vi "WSVCAP SHL Host LL Interface Manage Instance IDs.vi"(6 "Operation":T2, 8 "error in (no error)":errorcluster, 11 "FPGA":T3) -> (0 "error out":errorcluster, 3 "Instance IDs":T1)   [LabVIEW 2012]
uses:
  Type Defs/WSVCAP SHL I2C FPGA Enum.ctl
  user.lib/Utilities/Type Defs/MISC Instance Manager Operation.ctl
  Type Defs/WSVCAP SHL FPGA Interface Instance Ref Cluster.ctl
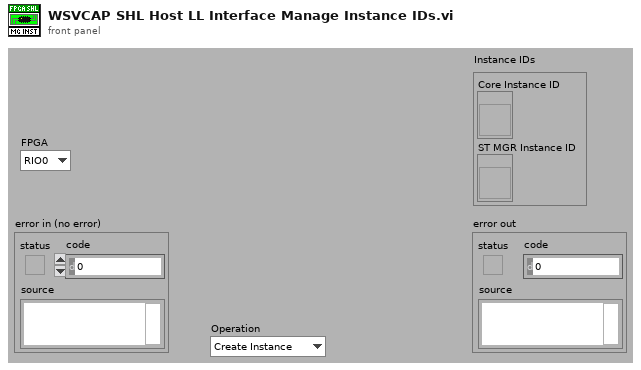
[diagram p1: front panel]
types:
  T1 = typedef "WSVCAP SHL FPGA Interface Instance Ref Cluster.ctl" = cluster{"Core Instance ID":refnum<vi>, "ST MGR Instance ID":refnum<vi>}
  T2 = typedef "MISC Instance Manager Operation.ctl" = enum16{"Create Instance", "Get Instance ID"}
  T3 = typedef "WSVCAP SHL I2C FPGA Enum.ctl" = enum16{"RIO0", "RIO1"}
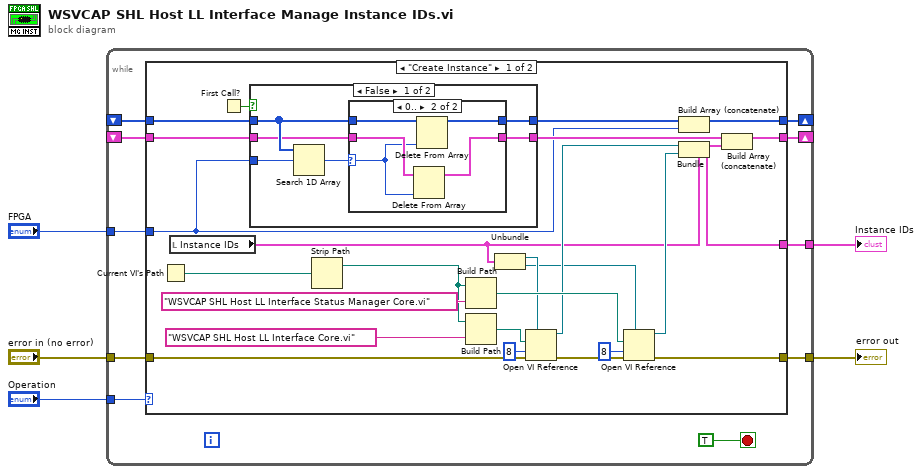
[diagram p0: block diagram]
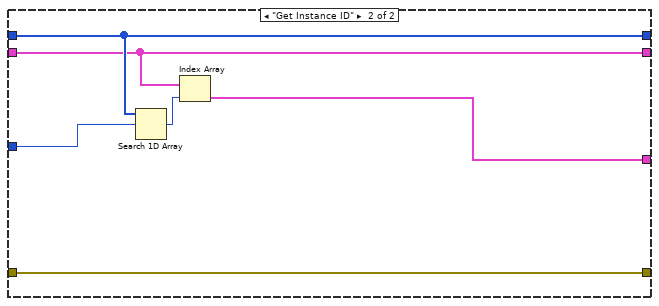
[diagram p4: hidden frame]
diagram:
  n1 = while {
    tunnel: "error in (no error)" -> [w15]
    tunnel: [w14] -> w4
    shift-right: [w8] -> _
    shift-left: _ -> [w11]
    shift-right: [w7] -> _
    shift-left: _ -> [w10]
    tunnel: "Operation" -> [w13]
    tunnel: "FPGA" -> [w9]
    tunnel: [w6] -> w1
    stop <- TRUE stop-if-true
    n2 = case shown="\"Create Instance\"" w13 {
      tunnel: w15 -> [w40 w55]
      tunnel: [w24 w55] -> w14
      tunnel: w11 -> [w37 w57]
      tunnel: w10 -> [w36 w56]
      tunnel: w9 -> [w33 w59]
      tunnel: [w39 w57] -> w8
      tunnel: [w29 w56] -> w7
      tunnel: [w20 w54] -> w6
      frame "Create Instance" {
        n3 = Current VI's Path() -> (path=w30:path)
        n4 = local read "Instance IDs"() -> (w19:T1)
        n5 = First Call?() -> (First Call?: T/F=w38:bool)
        n6 = case shown="False" w38 {
          tunnel: w37 -> [w45 _]
          tunnel: w36 -> [w44 _]
          tunnel: [w42 _] -> w35
          tunnel: [w41 _] -> w34
          tunnel: w33 -> [w46 _]
          frame False {
            n7 = Search 1D Array(1D array=w45, element=w46) -> (index of element=w43:i32)  [unwired: 1 out]
            n8 = case shown="0.." w43 {
              selector: w43 -> [_ w49]
              tunnel: w45 -> [w48 w53]
              tunnel: w44 -> [w47 w52]
              tunnel: [w48 w51] -> w42
              tunnel: [w47 w50] -> w41
              frame Default {
              }
              frame 0.. {
                n9 = Delete From Array(array=w52, index=w49) -> (array with subset deleted=w50:T1[])  [unwired: 1 in, 1 out]
                n10 = Delete From Array(array=w53, index=w49) -> (array with subset deleted=w51:T3[])  [unwired: 1 in, 1 out]
              }
            }
          }
          frame True {
          }
        }
        n11 = Strip Path(path=w30) -> (stripped path=w16:path)  [unwired: 1 out]
        n12 = Build Path(base path=w16, name or relative path="WSVCAP SHL Host LL Interface Status Manager Core.vi" ("vi path")) -> (appended path=w23:path)
        n13 = Build Path(base path=w16, name or relative path="WSVCAP SHL Host LL Interface Core.vi" ("vi path")) -> (appended path=w28:path)
        n14 = Unbundle(w19) -> ("Core Instance ID"=w18:refnum<vi>, "ST MGR Instance ID"=w17:refnum<vi>)
        n15 = Open VI Reference(type specifier VI Refnum (for type only)=w18, vi path=w28, options=8, error in (no error)=w40) -> (vi reference=w22:refnum<vi>, error out=w25:errorcluster)  [unwired: 2 out]
        n16 = Open VI Reference(type specifier VI Refnum (for type only)=w17, vi path=w23, options=8, error in (no error)=w25) -> (vi reference=w21:refnum<vi>, error out=w24:errorcluster)  [unwired: 2 out]
        n17 = Build Array (concatenate)(w35, w33) -> (w39:T3[])
        n18 = Bundle(cluster=w19, "Core Instance ID"=w22, "ST MGR Instance ID"=w21) -> (w20:T1)
        n19 = Build Array (concatenate)(w34, w20) -> (w29:T1[])
      }
      frame "Get Instance ID" {
        n20 = Search 1D Array(1D array=w57, element=w59) -> (index of element=w58:i32)  [unwired: 1 out]
        n21 = Index Array(array=w56, index=w58) -> (element=w54:T1)
      }
    }
  }
  "error out" <- w4
  "Instance IDs" <- w1
